vi "Motor_Trap.vi"() -> ()   [LabVIEW 2014]
uses:
  <vilib>/Simulation/Scripting/Companion Diagram/SimConfigNode/SimParams.ctl
  <vilib>/Simulation/Scripting/Companion Diagram/SimConfigNode/_simSolvers.ctl
  <vilib>/Simulation/Implementation/Shared/SIMSCR Execution Mode.ctl
  <vilib>/Simulation/Param Hierarchy/Typedefs/SIMPH Param Control Actions.ctl
  <vilib>/Simulation/Implementation/Shared/NILVSim_ParamChanged.vi
  <vilib>/Simulation/Implementation/Shared/NILVSIM_BeginStep.vi
  <vilib>/Simulation/DataSources/Implementation/NILVSim Step.llb/SIM Step (scalar).vi
  <vilib>/Simulation/Utility/Implementation/SIM Time.vi
  <vilib>/Simulation/Utility/Implementation/NILVSim Memory.llb/NILVSim Memory (core).vi
  <vilib>/Simulation/Utility/Implementation/NILVSim Collector.llb/SIM Collector (scalar).vi
  <vilib>/Simulation/SignalArithmetic/Implementation/NILVSim Gain.llb/SIM Gain (scalar).vi
  <vilib>/Simulation/Implementation/Shared/NILVSim_Manager.vi
  <vilib>/Utility/error.llb/Clear Errors.vi
  <vilib>/Simulation/Implementation/Shared/NILVSim_FinalizeModel.vi
  <vilib>/Simulation/Utility/Implementation/NILVSim Collector.llb/NILVSim Collector core (scalar).vi
  <vilib>/Simulation/Implementation/Shared/SIM Unbundle Sim Info.vi
  <vilib>/Simulation/Implementation/Shared/NILVSim_Initialize.vi
  <vilib>/Simulation/Utility/Implementation/NILVSim Get Time and IsAcceptedStep.vi
  Compute_trap_PID.vi
  <vilib>/Simulation/Implementation/Shared/SIMSH Read Queue.vi
  <vilib>/Simulation/Implementation/Shared/NILVSim_GetModelError.vi
  <vilib>/Simulation/Implementation/Shared/SIM Bundle Sim Info.vi
  <vilib>/Simulation/Scripting/Companion Diagram/SimConfigNode/SimDog.xnode
  <vilib>/Simulation/Implementation/XNodeFramework/SimXNode/SimX.xnode
  <vilib>/Simulation/EMI/Plugins/FMI for Model Exchange/EMI_FMIL.dll
  <vilib>/Simulation/Implementation/Shared/NI_SIM_Implementation.lvlib
panel:
  out "vProfile":cluster{"Time":dbl[], "Signal":dbl[]}(graph)
  in  "Acceleration [Rad/s^2]":dbl=100.0
  in  "Deceleration [Rad/s^2]":dbl=100.0
  in  "Vcruise [Rad/s]":dbl=200.0
  in  "MinFrac_Cruise":dbl=0.3
  in  "Kv":T1={"proportional gain (Kc)"=0.0006, "integral time (Ti, min)"=0.0005, "derivative time (Td, min)"=0.0} {"derivative time (Td, min)" format="%.1f"; "integral time (Ti, min)" format="%.1e"; "proportional gain (Kc)" format="%.1e"}
  in  "Kp":T1={"proportional gain (Kc)"=1.5, "integral time (Ti, min)"=0.0, "derivative time (Td, min)"=0.0} {"derivative time (Td, min)" format="%.1f"; "integral time (Ti, min)" format="%.1f"; "proportional gain (Kc)" format="%.1f"}
  out "Position [rad]":cluster{"Time":dbl[], "Signal":dbl[]}(graph)
  out "Velocity [rad/s]":cluster{"Time":dbl[], "Signal":dbl[]}(graph)
  out "Angular Velocity[rad/s]":dbl
  out "Position [rad]":dbl
  in  "Desired Position":dbl=1000.0
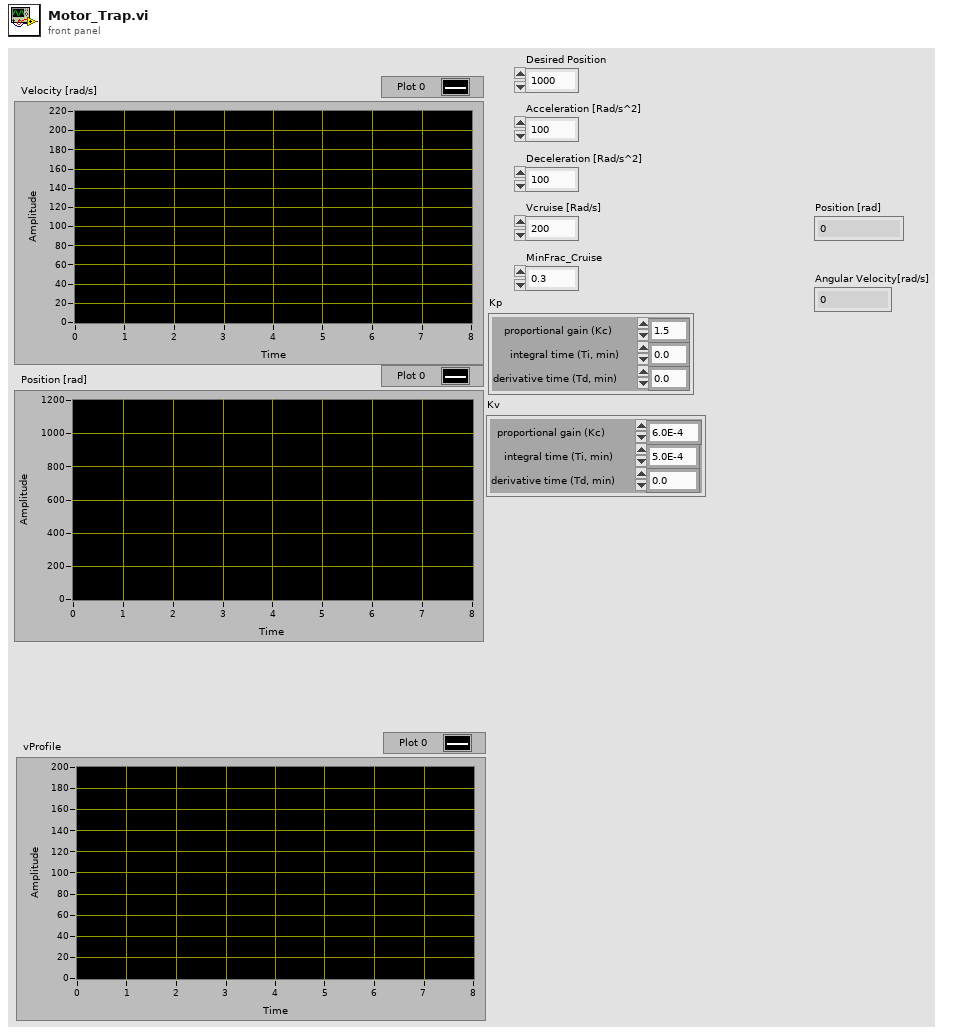
[diagram p1: front panel]
types:
  T1 = cluster{"proportional gain (Kc)":dbl, "integral time (Ti, min)":dbl, "derivative time (Td, min)":dbl}
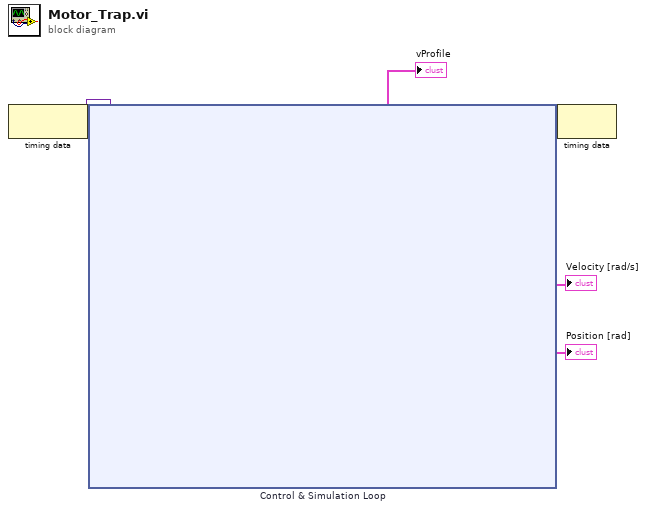
[diagram p0: block diagram]
diagram:
  n1 = node-c288() -> (w5:variant)  [unwired: 1 in]
  n2 = node-c254 "Control & Simulation Loop"(w5) -> (w4:variant, →"Velocity [rad/s]":cluster{"Time":dbl[], "Signal":dbl[]}, →"Position [rad]":cluster{"Time":dbl[], "Signal":dbl[]}, →"vProfile":cluster{"Time":dbl[], "Signal":dbl[]})
  n3 = node-c288(w4) -> ()  [unwired: 1 out]
